vi "MODUL 1 TESTING.vi"   [LabVIEW 2016, in "Test2.lvrbt"]
uses:
  Test2.lvrbt
  <vilib>/NXT/Hardware/Plugins/Tetrix DC Motor/TetrixDCMotorAddress.ctl
  <vilib>/NXT/Hardware/Plugins/Tetrix 180 deg Servo/Tetrix180ServoAddress.ctl
  <vilib>/NXT/Block Support/NXT_InputPort.ctl
  <vilib>/NXT/NXTIO Xnodes/NXTIONodeSubVIs/TETRIX IO Move Servos.vi
  <vilib>/NXT/Dual Mode Library/Waits/Wait_Num.vi
  <vilib>/NXT/NXTIO Xnodes/NXTIONodeSubVIs/TETRIX IO Move DC Motors.vi
  <vilib>/NXT/NXTIO Xnodes/NXTIONodeSubVIs/TETRIX IO Stop DC Motors.vi
  <vilib>/NXT/Dual Mode Library/Waits/Wait_EV3_Ultrasonic_Centimeter_Closer.vi
  <vilib>/NXT/Dual Mode Library/Waits/Wait_Touch.vi
  <vilib>/NXT/Dual Mode Library/Waits/Wait_EV3_Ultrasonic_Centimeters_Further.vi
  <vilib>/NXT/NXTIO Xnodes/AddressXNode/NXTIOAddress.xnode
  <vilib>/NXT/Subs/LVHSConnector.ctl
  <vilib>/NXT/NXTIO Xnodes/NXTIOXNode/NXTIO.xnode
  <vilib>/NXT/LegoClasses/BrickReference/BrickReference.lvclass
types:
  T1 = typedef "Tetrix180ServoAddress.ctl" = i32
  T2 = cluster{"Tetrix180Servo":T1, "Tetrix180Servo 2":T1, "Tetrix180Servo 3":T1, "Tetrix180Servo 4":T1, "Tetrix180Servo 5":T1, "Tetrix180Servo 6":T1}
  T3 = typedef "TetrixDCMotorAddress.ctl" = i32
  T4 = cluster{"TetrixDCMotor":T3, "TetrixDCMotor 2":T3}
  T5 = cluster{"Tetrix180Servo":T1, "Tetrix180Servo":T1, "Tetrix180Servo":T1, "Tetrix180Servo":T1, "Tetrix180Servo":T1, "Tetrix180Servo":T1}
  T6 = typedef "LVHSConnector.ctl" = refnum<class "BrickReference.lvclass">
  T7 = typedef "NXT_InputPort.ctl" = u32
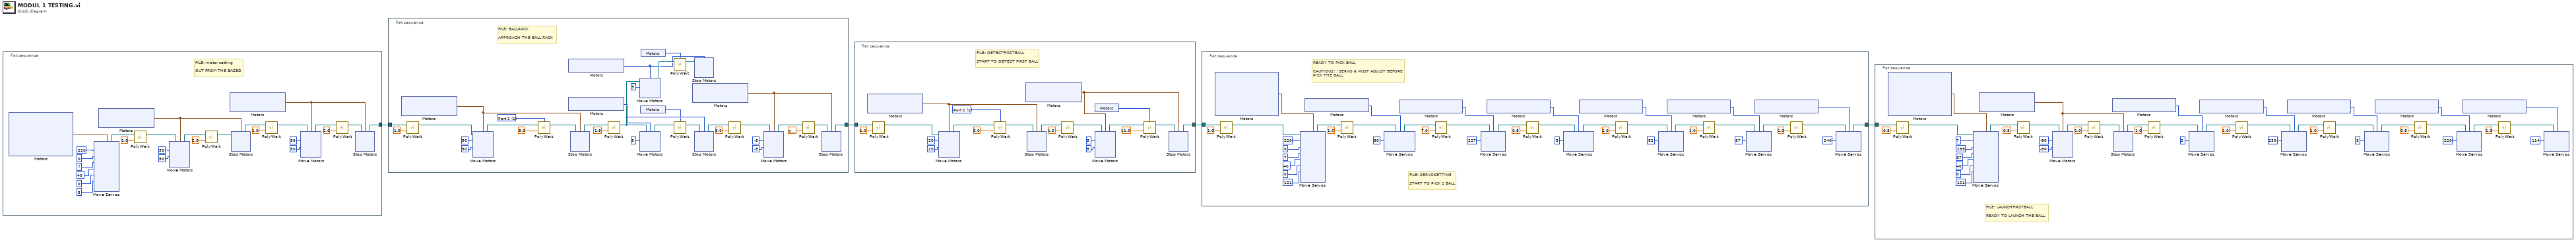
[diagram p0: block diagram]
diagram:
  n1 = flat-sequence {
    tunnel: [w15] -> w4
    frame #0 {
      # "FILE: motor setting\n\nOUT FROM THE BASED"
      n2 = xnode "Motors"() -> ("Motor"=w14:T5)
      n3 = xnode "Move Servos"("Position 6"=u8 5, "Position 5"=u8 0, "Position 4"=u8 40, "Position 3"=u8 7, "Position 2"=u8 0, "Position 1"=u8 220, "Motors"=w14) -> ("NXT/EV3"=w12:T6)  [unwired: 1 in]
      n4 = xnode "Motors"() -> ("Motor"=w19:cluster{"TetrixDCMotor":T3, "TetrixDCMotor":T3})
      n5 = call-poly <vilib>:"PolyWait.vi"("Time (1 sec)"=sgl 1.0, "NXT/EV3"=w12) -> ("NXT/EV3"=w11:T6)  [unwired: 2 in]
      n6 = xnode "Move Motors"("Power/Speed 2"=i8 50, "Power/Speed 1"=i8 50, "Motors"=w19, "NXT/EV3"=w11) -> ("NXT/EV3"=w22:T6)
      n7 = call-poly <vilib>:"PolyWait.vi"("Time (1 sec)"=sgl 2.0, "NXT/EV3"=w22) -> ("NXT/EV3"=w20:T6)  [unwired: 2 in]
      n8 = xnode "Motors"() -> ("Motor"=w25:cluster{"TetrixDCMotor":T3, "TetrixDCMotor":T3})
      n9 = xnode "Stop Motors"("Motors"=w19, "NXT/EV3"=w20) -> ("NXT/EV3"=w18:T6)
      n10 = call-poly <vilib>:"PolyWait.vi"("Time (1 sec)"=sgl 1.0, "NXT/EV3"=w18) -> ("NXT/EV3"=w16:T6)  [unwired: 2 in]
      n11 = xnode "Move Motors"("Power/Speed 2"=i8 50, "Power/Speed 1"=i8 50, "Motors"=w25, "NXT/EV3"=w16) -> ("NXT/EV3"=w28:T6)
      n12 = call-poly <vilib>:"PolyWait.vi"("Time (1 sec)"=sgl 2.0, "NXT/EV3"=w28) -> ("NXT/EV3"=w26:T6)  [unwired: 2 in]
      n13 = xnode "Stop Motors"("Motors"=w25, "NXT/EV3"=w26) -> ("NXT/EV3"=w15:T6)
    }
  }
  n14 = flat-sequence {
    tunnel: w4 -> [w74]
    tunnel: [w72] -> w3
    frame #0 {
      w85 = T7 1 items=["Port 1", "Port 2", "Port 3", "Port 4"] ("Port (Port 1)")
      # "FILE: BALLRACK\n\nAPPROACH THE BALL RACK"
      n15 = xnode "Motors"() -> ("Motor"=w99:cluster{"TetrixDCMotor":T3, "TetrixDCMotor":T3})
      n16 = call-poly <vilib>:"PolyWait.vi"("Time (1 sec)"=sgl 1.0, "NXT/EV3"=w74) -> ("NXT/EV3"=w73:T6)  [unwired: 2 in]
      n17 = xnode "Move Motors"("Power/Speed 2"=i8 50, "Power/Speed 1"=i8 50, "Motors"=w99, "NXT/EV3"=w73) -> ("NXT/EV3"=w102:T6)
      n18 = call-poly <vilib>:"PolyWait.vi"("Centimeters (40)"=sgl 8.0, "NXT/EV3"=w102, "Port (Port 1)"=w85) -> ("NXT/EV3"=w100:T6)  [unwired: 1 in]
      n19 = xnode "Motors"() -> ("Motor"=w95:T3)
      n20 = xnode "Motors"() -> ("Motor"=w90:T3)
      n21 = xnode "Stop Motors"("Motors"=w99, "NXT/EV3"=w100) -> ("NXT/EV3"=w93:T6)
      n22 = call-poly <vilib>:"PolyWait.vi"("Time (1 sec)"=sgl 1.5, "NXT/EV3"=w93) -> ("NXT/EV3"=w88:T6)  [unwired: 2 in]
      n23 = xnode "Move Motors"("Power/Speed 1"=i8 5, "Motors"=w95, "NXT/EV3"=w88) -> ("NXT/EV3"=w97:T6)
      n24 = xnode "Move Motors"("Power/Speed 1"=i8 5, "Motors"=w90, "NXT/EV3"=w88) -> ("NXT/EV3"=w91:T6)
      n25 = xnode "Motors"() -> ("Sensor"=w87:T7)
      n26 = xnode "Motors"() -> ("Sensor"=w86:T7)
      n27 = call-poly <vilib>:"PolyWait.vi"("NXT/EV3"=w97, "Port (Port 1)"=w86) -> ("NXT/EV3"=w96:T6)  [unwired: 2 in]
      n28 = call-poly <vilib>:"PolyWait.vi"("NXT/EV3"=w91, "Port (Port 1)"=w87) -> ("NXT/EV3"=w89:T6)  [unwired: 2 in]
      n29 = xnode "Motors"() -> ("Motor"=w82:cluster{"TetrixDCMotor":T3, "TetrixDCMotor":T3})
      n30 = xnode "Stop Motors"("Motors"=w95, "NXT/EV3"=w96) -> ()  [unwired: 1 out]
      n31 = xnode "Stop Motors"("Motors"=w90, "NXT/EV3"=w89) -> ("NXT/EV3"=w84:T6)
      n32 = call-poly <vilib>:"PolyWait.vi"("Time (1 sec)"=sgl 3.0, "NXT/EV3"=w84) -> ("NXT/EV3"=w80:T6)  [unwired: 2 in]
      n33 = xnode "Move Motors"("Power/Speed 2"=i8 -5, "Power/Speed 1"=i8 -5, "Motors"=w82, "NXT/EV3"=w80) -> ("NXT/EV3"=w77:T6)
      n34 = call-poly <vilib>:"PolyWait.vi"("Time (1 sec)"=sgl 0.2, "NXT/EV3"=w77) -> ("NXT/EV3"=w76:T6)  [unwired: 2 in]
      n35 = xnode "Stop Motors"("Motors"=w82, "NXT/EV3"=w76) -> ("NXT/EV3"=w72:T6)
    }
  }
  n36 = flat-sequence {
    tunnel: w3 -> [w180]
    tunnel: [w161] -> w2
    frame #0 {
      w176 = T7 1 items=["Port 1", "Port 2", "Port 3", "Port 4"] ("Port (Port 1)")
      # "FILE: DETECTFIRSTBALL\n\nSTART TO DETECT FIRST BALL"
      n37 = xnode "Motors"() -> ("Motor"=w173:cluster{"TetrixDCMotor":T3, "TetrixDCMotor":T3})
      n38 = call-poly <vilib>:"PolyWait.vi"("Time (1 sec)"=sgl 1.0, "NXT/EV3"=w180) -> ("NXT/EV3"=w162:T6)  [unwired: 2 in]
      n39 = xnode "Move Motors"("Power/Speed 2"=i8 20, "Power/Speed 1"=i8 20, "Motors"=w173, "NXT/EV3"=w162) -> ("NXT/EV3"=w179:T6)
      n40 = call-poly <vilib>:"PolyWait.vi"("Centimeters (50)"=sgl 6.0, "NXT/EV3"=w179, "Port (Port 1)"=w176) -> ("NXT/EV3"=w177:T6)  [unwired: 1 in]
      n41 = xnode "Motors"() -> ("Motor"=w169:cluster{"TetrixDCMotor":T3, "TetrixDCMotor":T3})
      n42 = xnode "Stop Motors"("Motors"=w173, "NXT/EV3"=w177) -> ("NXT/EV3"=w163:T6)
      n43 = call-poly <vilib>:"PolyWait.vi"("Time (1 sec)"=sgl 1.0, "NXT/EV3"=w163) -> ("NXT/EV3"=w164:T6)  [unwired: 2 in]
      n44 = xnode "Move Motors"("Power/Speed 2"=i8 5, "Power/Speed 1"=i8 5, "Motors"=w169, "NXT/EV3"=w164) -> ("NXT/EV3"=w171:T6)
      n45 = xnode "Motors"() -> ("Sensor"=w166:T7)
      n46 = call-poly <vilib>:"PolyWait.vi"("Centimeters (40)"=sgl 11.0 ("Centimeters (50)"), "NXT/EV3"=w171, "Port (Port 1)"=w166) -> ("NXT/EV3"=w170:T6)  [unwired: 1 in]
      n47 = xnode "Stop Motors"("Motors"=w169, "NXT/EV3"=w170) -> ("NXT/EV3"=w161:T6)
    }
  }
  n48 = flat-sequence {
    tunnel: w2 -> [w250]
    tunnel: [w211] -> w1
    frame #0 {
      # "READY TO PICK BALL\n\nCAUTIOUS! : SERVO 6 MUST ADJUST BEFORE\nPICK THE BALL"
      # "FILE: SERVOSETTING\n\nSTART TO PICK 1 BALL"
      n49 = xnode "Motors"() -> ("Motor"=w237:T5)
      n50 = call-poly <vilib>:"PolyWait.vi"("Time (1 sec)"=sgl 1.0, "NXT/EV3"=w250) -> ("NXT/EV3"=w213:T6)  [unwired: 2 in]
      n51 = xnode "Move Servos"("Position 6"=u8 121, "Position 5"=u8 0, "Position 4"=u8 40, "Position 3"=u8 7, "Position 2"=u8 0, "Position 1"=u8 220, "Motors"=w237, "NXT/EV3"=w213) -> ("NXT/EV3"=w212:T6)
      n52 = xnode "Motors"() -> ("Motor"=w249:T1)
      n53 = call-poly <vilib>:"PolyWait.vi"("Time (1 sec)"=sgl 1.0, "NXT/EV3"=w212) -> ("NXT/EV3"=w225:T6)  [unwired: 2 in]
      n54 = xnode "Move Servos"("Position 1"=u8 60, "Motors"=w249, "NXT/EV3"=w225) -> ("NXT/EV3"=w246:T6)
      n55 = xnode "Motors"() -> ("Motor"=w245:T1)
      n56 = call-poly <vilib>:"PolyWait.vi"("Time (1 sec)"=sgl 7.0, "NXT/EV3"=w246) -> ("NXT/EV3"=w243:T6)  [unwired: 2 in]
      n57 = xnode "Move Servos"("Position 1"=u8 227, "Motors"=w245, "NXT/EV3"=w243) -> ("NXT/EV3"=w241:T6)
      n58 = xnode "Motors"() -> ("Motor"=w240:T1)
      n59 = call-poly <vilib>:"PolyWait.vi"("Time (1 sec)"=sgl 0.5, "NXT/EV3"=w241) -> ("NXT/EV3"=w238:T6)  [unwired: 2 in]
      n60 = xnode "Move Servos"("Position 1"=u8 5, "Motors"=w240, "NXT/EV3"=w238) -> ("NXT/EV3"=w230:T6)
      n61 = xnode "Motors"() -> ("Motor"=w228:T1)
      n62 = call-poly <vilib>:"PolyWait.vi"("Time (1 sec)"=sgl 1.0, "NXT/EV3"=w230) -> ("NXT/EV3"=w227:T6)  [unwired: 2 in]
      n63 = xnode "Move Servos"("Position 1"=u8 82, "Motors"=w228, "NXT/EV3"=w227) -> ("NXT/EV3"=w214:T6)
      n64 = xnode "Motors"() -> ("Motor"=w222:T1)
      n65 = call-poly <vilib>:"PolyWait.vi"("Time (1 sec)"=sgl 1.0, "NXT/EV3"=w214) -> ("NXT/EV3"=w221:T6)  [unwired: 2 in]
      n66 = xnode "Move Servos"("Position 1"=u8 67, "Motors"=w222, "NXT/EV3"=w221) -> ("NXT/EV3"=w219:T6)
      n67 = xnode "Motors"() -> ("Motor"=w217:T1)
      n68 = call-poly <vilib>:"PolyWait.vi"("Time (1 sec)"=sgl 1.0, "NXT/EV3"=w219) -> ("NXT/EV3"=w216:T6)  [unwired: 2 in]
      n69 = xnode "Move Servos"("Position 1"=u8 240, "Motors"=w217, "NXT/EV3"=w216) -> ("NXT/EV3"=w211:T6)
    }
  }
  n70 = flat-sequence {
    tunnel: w1 -> [w355]
    frame #0 {
      # "FILE: LAUNCHFIRSTBALL \n\nREADY TO LAUNCH THE BALL"
      n71 = xnode "Motors"() -> ("Motor"=w348:T5)
      n72 = call-poly <vilib>:"PolyWait.vi"("Time (1 sec)"=sgl 0.5, "NXT/EV3"=w355) -> ("NXT/EV3"=w313:T6)  [unwired: 2 in]
      n73 = xnode "Move Servos"("Position 6"=u8 121, "Position 5"=u8 0, "Position 4"=u8 40, "Position 3"=u8 67, "Position 2"=u8 255, "Position 1"=u8 7, "Motors"=w348, "NXT/EV3"=w313) -> ("NXT/EV3"=w340:T6)
      n74 = xnode "Motors"() -> ("Motor"=w349:cluster{"TetrixDCMotor":T3, "TetrixDCMotor":T3})
      n75 = call-poly <vilib>:"PolyWait.vi"("Time (1 sec)"=sgl 0.5, "NXT/EV3"=w340) -> ("NXT/EV3"=w339:T6)  [unwired: 2 in]
      n76 = xnode "Move Motors"("Power/Speed 2"=i8 -50, "Power/Speed 1"=i8 -50, "Motors"=w349, "NXT/EV3"=w339) -> ("NXT/EV3"=w352:T6)
      n77 = call-poly <vilib>:"PolyWait.vi"("Time (1 sec)"=sgl 1.0, "NXT/EV3"=w352) -> ("NXT/EV3"=w350:T6)  [unwired: 2 in]
      n78 = xnode "Motors"() -> ("Motor"=w335:T1)
      n79 = xnode "Stop Motors"("Motors"=w349, "NXT/EV3"=w350) -> ("NXT/EV3"=w338:T6)
      n80 = call-poly <vilib>:"PolyWait.vi"("Time (1 sec)"=sgl 1.0, "NXT/EV3"=w338) -> ("NXT/EV3"=w336:T6)  [unwired: 2 in]
      n81 = xnode "Move Servos"("Position 1"=u8 0, "Motors"=w335, "NXT/EV3"=w336) -> ("NXT/EV3"=w329:T6)
      n82 = xnode "Motors"() -> ("Motor"=w331:T1)
      n83 = call-poly <vilib>:"PolyWait.vi"("Time (1 sec)"=sgl 1.0, "NXT/EV3"=w329) -> ("NXT/EV3"=w332:T6)  [unwired: 2 in]
      n84 = xnode "Move Servos"("Position 1"=u8 230, "Motors"=w331, "NXT/EV3"=w332) -> ("NXT/EV3"=w324:T6)
      n85 = xnode "Motors"() -> ("Motor"=w326:T1)
      n86 = call-poly <vilib>:"PolyWait.vi"("Time (1 sec)"=sgl 1.0, "NXT/EV3"=w324) -> ("NXT/EV3"=w327:T6)  [unwired: 2 in]
      n87 = xnode "Move Servos"("Position 1"=u8 5, "Motors"=w326, "NXT/EV3"=w327) -> ("NXT/EV3"=w319:T6)
      n88 = xnode "Motors"() -> ("Motor"=w321:T1)
      n89 = call-poly <vilib>:"PolyWait.vi"("Time (1 sec)"=sgl 0.5, "NXT/EV3"=w319) -> ("NXT/EV3"=w322:T6)  [unwired: 2 in]
      n90 = xnode "Move Servos"("Position 1"=u8 220, "Motors"=w321, "NXT/EV3"=w322) -> ("NXT/EV3"=w314:T6)
      n91 = xnode "Motors"() -> ("Motor"=w316:T1)
      n92 = call-poly <vilib>:"PolyWait.vi"("Time (1 sec)"=sgl 1.0, "NXT/EV3"=w314) -> ("NXT/EV3"=w317:T6)  [unwired: 2 in]
      n93 = xnode "Move Servos"("Position 1"=u8 114, "Motors"=w316, "NXT/EV3"=w317) -> ()  [unwired: 1 out]
    }
  }
